vi "Create Symbol Information Loader.vi"(8 "error in (no error)":errorcluster, 11 "TwinCAT ADS in":refnum<class "TwinCAT ADS.lvclass">) -> (0 "error out":errorcluster, 3 "TwinCAT ADS out":refnum<class "TwinCAT ADS.lvclass">)   [LabVIEW 2018, in "TwinCAT ADS.lvclass"]
uses:
  TwinCAT ADS.lvclass
  TwinCAT ADS.lvclass/TwinCAT ADS.ctl
  TwinCAT.Ads
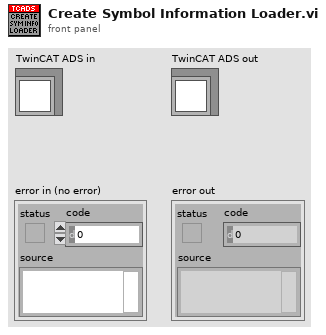
[diagram p1: front panel]
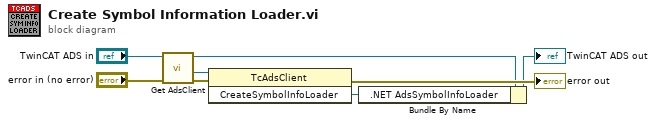
[diagram p0: block diagram]
diagram:
  n1 = call "Get AdsClient.vi"("error in (no error)"="error in (no error)", "TwinCAT ADS in"="TwinCAT ADS in") -> ("error out"=w5:errorcluster, ".NET TcAdsClient"=w4:refnum<k24>, "TwinCAT ADS out"=w3:refnum<class "TwinCAT ADS.lvclass">)  [unwired: 7 in]
  n2 = invoke class="TcAdsClient" method="CreateSymbolInfoLoader"(reference=w4, error in=w5) -> (error out=→"error out":errorcluster, "CreateSymbolInfoLoader"=w2:refnum<k24>)  [unwired: 1 in, 1 out]
  n3 = Bundle By Name(cluster=w3, ".NET AdsSymbolInfoLoader"=w2) -> (→"TwinCAT ADS out":refnum<class "TwinCAT ADS.lvclass">)
